vi "Monitor B Variable.vi"() -> ()   [LabVIEW 2012]
panel:
  out "Monitor B Array":dbl[](array[numeric])
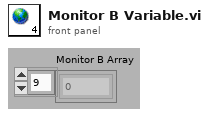
[diagram p1: front panel]
diagram:
